vi "test_json_decoder.vi"() -> ()   [LabVIEW 2019]
doc: "JSON VI Tree.\n\nCreated by: Ryan Pacini"
uses:
  json/JSON.lvlib
panel:
  out "Filename":string
  out "Iter":i32
  out "Count":i32
  out "test cases":T1(array[cluster])
  in  "JSON test dir":path=path "C:/Projects/git/labview_json/tests/JSONTestSuite/test_parsing"
  # "https://github.com/nst/JSONTestSuite"
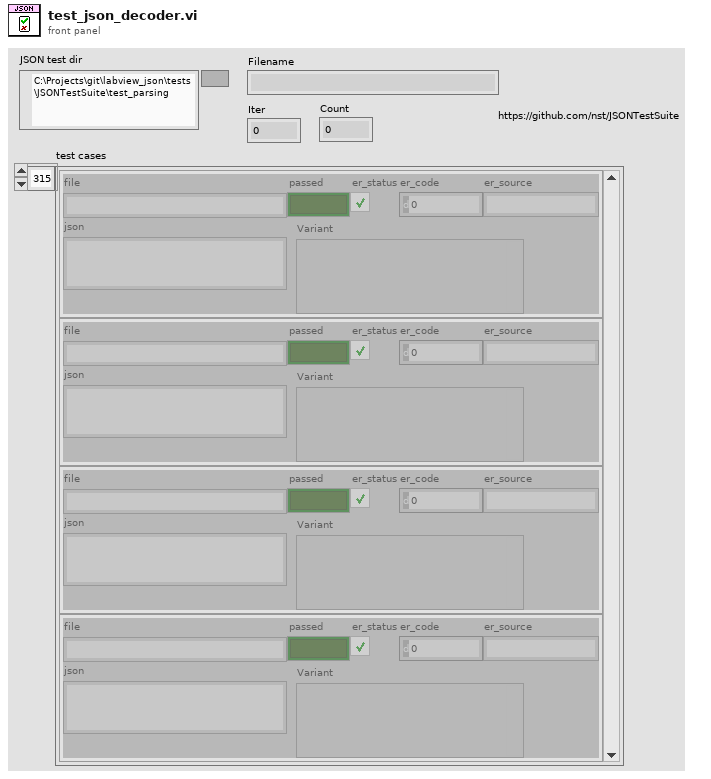
[diagram p1: front panel]
types:
  T1 = cluster{"file":string, "json":string, "Variant":variant, "passed":bool, "er_status":bool, "er_code":i32, "er_source":string}[]
  T2 = cluster{"file":string, "json":string, variant, "passed":bool, "er_status":bool, "er_code":i32, "er_source":string}[]
  T3 = cluster{string, string, "Variant out":variant, "status":bool, "status":bool, "code":i32, "source":string}
  T4 = cluster{"file":string, "json":string, "Variant out":variant, "status":bool, "status":bool, "code":i32, "source":string}[]
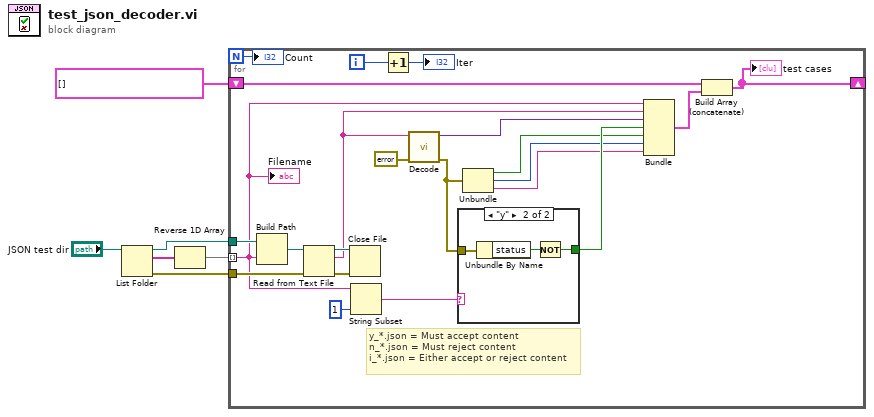
[diagram p0: block diagram]
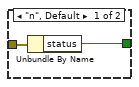
[diagram p2: hidden frame]
diagram:
  n1 = List Folder(path="JSON test dir") -> (path out=w4:path, filenames=w3:string[], error out=w5:errorcluster)  [unwired: 3 in, 1 out]
  n2 = Reverse 1D Array(array=w3) -> (reversed array=w1:string[])
  n3 = for {
    N -> [w10]
    tunnel: w5 -> [w28]
    tunnel: w4 -> [w26]
    tunnel: w1 -> [w22] mode=indexing
    shift-right: [w11] -> _
    shift-left: T2 [] ("test cases") -> [w13]
    i -> [w9]
    # "y_*.json = Must accept content\nn_*.json = Must reject content\ni_*.json = Either accept or reject content"
    n4 = Build Path(base path=w26, name or relative path=w22) -> (appended path=w25:path)
    n5 = Read from Text File(file (use dialog)=w25, error in=w28) -> (refnum out=w24:refnum<file>, text=w23:string, error out=w27:errorcluster)  [unwired: 2 in, 1 out]
    n6 = Close File(refnum=w24, error in=w27) -> ()  [unwired: 2 out]
    n7 = String Subset(string=w22, length (rest)=1 ("length (rest)")) -> (substring=w19:string)  [unwired: 1 in]
    n8 = Increment(x=w9) -> (x+1=→"Iter":i32)
    n9 = call "Decode.vi"("error in (no error)"=errorcluster {"status"=FALSE, "code"=0, "source"=""}, "JSON in"=w23) -> ("error out"=w17:errorcluster, "Variant out"=w8:variant)  [unwired: 8 in]
    n10 = case shown="\"y\"" w19 {
      tunnel: w17 -> [w30 w33]
      tunnel: [w29 w31] -> w18
      frame "n", Default {
        n11 = Unbundle By Name(w30) -> ("status"=w29:bool)
      }
      frame "y" {
        n12 = Unbundle By Name(w33) -> ("status"=w32:bool)
        n13 = Not(x=w32) -> (.not. x?=w31:bool)
      }
    }
    n14 = Unbundle(w17) -> ("status"=w16:bool, "code"=w15:i32, "source"=w14:string)
    n15 = Bundle(w22, w23, "Variant out"=w8, "status"=w18, "status"=w16, "code"=w15, "source"=w14) -> (w12:T3)  [unwired: 1 in]
    n16 = Build Array (concatenate)(w13, w12) -> (w11:T4)
    "test cases" <- w11
    "Count" <- w10
    "Filename" <- w22
  }
